vi "Calibrate Drive.vi"(0 "Initiate Calibration":bool) -> (1 "Counts":i32, 2 "Time (ms)":u32)   [LabVIEW 2013]
uses:
  <vilib>/Rock Robotics/WPI/RobotDrive/WPI_RobotDriveMecanumDrive_Cartesian.vi
panel:
  in  "Acceleration Time (ms)":u32
  in  "Motor Speed":dbl
  out "Start Time":u32
  in  "Max Stopped Period":dbl
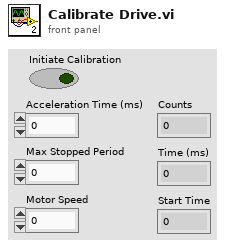
[diagram p1: front panel]
types:
  T1 = typedef "WPI_CounterDevRef.ctl" = cluster{"DevStatus":errorcluster, "CntIndex":T2}
  T2 = typedef "FPGA_CounterCtrSystemIndex.ctl" = enum8{"Ctr 0", "Ctr 1", "Ctr 2", "Ctr 3", "Ctr 4", "Ctr 5", "Ctr 6", "Ctr 7", "Invalid"}
  T3 = typedef "WPI_RobotDriveDevRef.ctl" = cluster{"DevStatus":errorcluster, "Motors[]":T4[], "Square Inputs":bool, "Max Output":dbl, "Isochronous":bool}
  T4 = typedef "WPI_MotorControlDeviceRef.ctl" = cluster{"DeviceStatus":errorcluster, "Type":enum16{"PWM", "CAN"}, "PWM":cluster{"Digital Module":T5, "PWM Channel":T6, "DeadBand":T7}, "CAN":cluster{"Device Number":u8, "Control Mode":T8, "Semaphore":T9, "Max Vout":dbl}, "Invert":bool, "TransformRef":T10, "InvTransformRef":T10}
  T5 = typedef "FPGA_TypedefDigitalModule.ctl" = enum16{"Digital Module 1", "Digital Module 2"}
  T6 = typedef "FPGA_DIOPWMChannel.ctl" = enum8{"PWM 1", "PWM 2", "PWM 3", "PWM 4", "PWM 5", "PWM 6", "PWM 7", "PWM 8", "PWM 9", "PWM 10", "Invalid"}
  T7 = typedef "WPI_PWMDeadband.ctl" = cluster{"Name":string, "maxPositivePwm":i32, "minPositivePwm":i32, "centerPwm":i32, "maxNegativePwm":i32, "minNegativePwm":i32, "angularRange":u16}
  T8 = typedef "WPI_CANJaguar_ControlMode.ctl" = enum8{"Percent VBus", "Current", "Speed", "Position", "Voltage"}
  T9 = typedef "Semaphore RefNum" = refnum<k1>
  T10 = typedef "WPI_PWMTransform_ConPane.ctl" = refnum<vi>
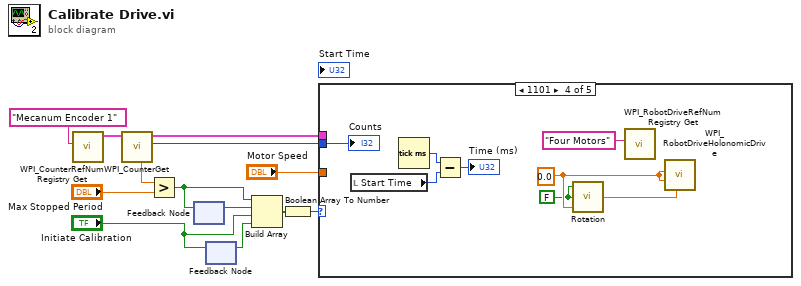
[diagram p0: block diagram]
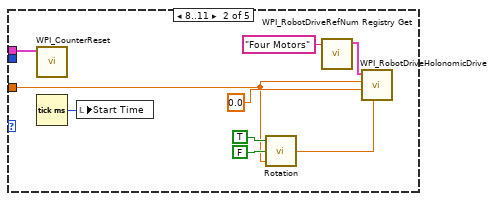
[diagram p3: hidden frame]
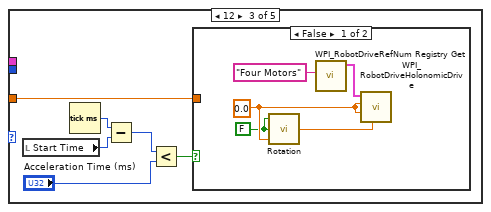
[diagram p4: hidden frame]
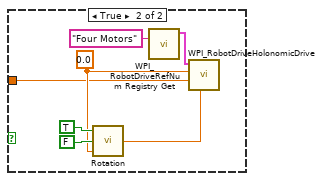
[diagram p5: hidden frame]
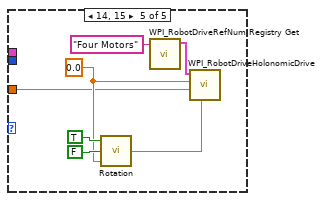
[diagram p6: hidden frame]
diagram:
  n1 = call <vilib>:"WPI_CounterRefNum Registry Get.vi"("refnum name"="Mecanum Encoder 1") -> ("CounterDevRef"=w11:T1)  [unwired: 9 in, 1 out]
  n2 = call <vilib>:"WPI_CounterGet.vi"("CounterDevRef in"=w11) -> ("Value"=w8:i32, "CounterDevRef out"=w9:T1, "Period (sec)"=w10:dbl)  [unwired: 5 in, 3 out]
  n3 = Greater?(x=w10, y="Max Stopped Period") -> (0:w2:bool)
  n4 = feedback #1() -> (w3:bool)  [unwired: 1 in]
  n5 = feedback-in #1(w2) -> ()
  n6 = feedback-in #2("Initiate Calibration") -> ()
  n7 = feedback #2() -> (w4:bool)  [unwired: 1 in]
  n8 = Build Array(w2, w3, "Initiate Calibration", w4) -> (w5:bool[])
  n9 = Boolean Array To Number(Boolean array=w5) -> (number=w6:u32)
  n10 = case shown="1101" w6 {
    tunnel: w9 -> [_ w15 _ _ _]
    tunnel: w8 -> [_ _ _ w43 _]
    tunnel: "Motor Speed" -> [_ w14 w23 _ w49]
    frame 0..7 {
    }
    frame 8..11 {
      n11 = call <vilib>:"WPI_CounterReset.vi"("CounterDevRef in"=w15) -> ()  [unwired: 9 in, 2 out]
      n12 = Tick Count (ms)() -> (millisecond timer value=w22:u32)
      n13 = local write "Start Time"(w22) -> ()
      n14 = call "Rotation.vi"("Uncorrected Speed"=w14, "Rotating Manually"=FALSE, "Moving Laterally"=TRUE) -> ("Output Speed"=w18:dbl)
      n15 = call <vilib>:"WPI_RobotDriveRefNum Registry Get.vi"("refnum name"="Four Motors") -> ("RobotDriveDevRef"=w16:T3)  [unwired: 1 in, 9 out]
      n16 = call-poly <vilib>:"WPI_RobotDriveHolonomicDrive.vi"("Rotation"=w18, "Y"=0.0, "X"=w14, "RobotDriveDevRef"=w16) -> ()  [unwired: 5 in, 3 out]
    }
    frame 12 {
      n17 = local read "Start Time"() -> (w27:u32)
      n18 = Tick Count (ms)() -> (millisecond timer value=w28:u32)
      n19 = Subtract(x=w28, y=w27) -> (x-y=w25:u32)
      n20 = Less?(x=w25, y="Acceleration Time (ms)") -> (x < y?=w26:bool)
      n21 = case shown="False" w26 {
        tunnel: w23 -> [_ w34]
        frame False {
          w31 = 0.0
          w30 = FALSE
          n22 = call "Rotation.vi"("Uncorrected Speed"=w31, "Rotating Manually"=w30, "Moving Laterally"=w30) -> ("Output Speed"=w32:dbl)
          n23 = call <vilib>:"WPI_RobotDriveRefNum Registry Get.vi"("refnum name"="Four Motors") -> ("RobotDriveDevRef"=w29:T3)  [unwired: 1 in, 9 out]
          n24 = call-poly <vilib>:"WPI_RobotDriveHolonomicDrive.vi"("Rotation"=w32, "Y"=w31, "X"=w31, "RobotDriveDevRef"=w29) -> ()  [unwired: 5 in, 3 out]
        }
        frame True {
          w35 = 0.0
          n25 = call "Rotation.vi"("Uncorrected Speed"=w35, "Rotating Manually"=FALSE, "Moving Laterally"=TRUE) -> ("Output Speed"=w38:dbl)
          n26 = call <vilib>:"WPI_RobotDriveRefNum Registry Get.vi"("refnum name"="Four Motors") -> ("RobotDriveDevRef"=w36:T3)  [unwired: 1 in, 9 out]
          n27 = call-poly <vilib>:"WPI_RobotDriveHolonomicDrive.vi"("Rotation"=w38, "Y"=w34, "X"=w35, "RobotDriveDevRef"=w36) -> ()  [unwired: 5 in, 3 out]
        }
      }
    }
    frame 13 {
      w44 = 0.0
      w41 = FALSE
      n28 = local read "Start Time"() -> (w42:u32)
      n29 = Tick Count (ms)() -> (millisecond timer value=w48:u32)
      n30 = Subtract(x=w48, y=w42) -> (x-y=→"Time (ms)":u32)
      n31 = call "Rotation.vi"("Uncorrected Speed"=w44, "Rotating Manually"=w41, "Moving Laterally"=w41) -> ("Output Speed"=w45:dbl)
      n32 = call <vilib>:"WPI_RobotDriveRefNum Registry Get.vi"("refnum name"="Four Motors") -> ()  [unwired: 1 in, 10 out]
      n33 = call-poly <vilib>:"WPI_RobotDriveHolonomicDrive.vi"("Rotation"=w45, "Y"=w44, "X"=w44) -> ()  [unwired: 6 in, 3 out]
      "Counts" <- w43
    }
    frame 14, 15 {
      w50 = 0.0
      n34 = call "Rotation.vi"("Uncorrected Speed"=w50, "Rotating Manually"=FALSE, "Moving Laterally"=TRUE) -> ("Output Speed"=w53:dbl)
      n35 = call <vilib>:"WPI_RobotDriveRefNum Registry Get.vi"("refnum name"="Four Motors") -> ("RobotDriveDevRef"=w51:T3)  [unwired: 1 in, 9 out]
      n36 = call-poly <vilib>:"WPI_RobotDriveHolonomicDrive.vi"("Rotation"=w53, "Y"=w49, "X"=w50, "RobotDriveDevRef"=w51) -> ()  [unwired: 5 in, 3 out]
    }
  }
